vi "enumerateStaticDependencies.vi"(8 "error in (no error)":errorcluster, 11 "SMO.A":refnum<class "SMO.A.lvclass">) -> (0 "error out":errorcluster, 2 "Static Dependencies":refnum<class "SMODependency.lvclass">[](array[class]), 3 "SMO.A out":refnum<class "SMO.A.lvclass">)   [LabVIEW 2013, in "SMO.A.lvclass"]
uses:
  SMO.A.lvclass
  src/Dependency/SMODependency.lvclass
  src/SMO/SMO.lvclass
panel:
  # "For instructions on how to use the JKI State Machine Objects, examples and video tutorials, visit:\nhttp://jki.net/state-machine-objects/\n\nJKI State Machine Objects™\nhttp://jki.net/state-machine-objects/\nCopyright (C) 2005-2015, JKI <info@jki.net>\nALL RIGHTS RESERVED"
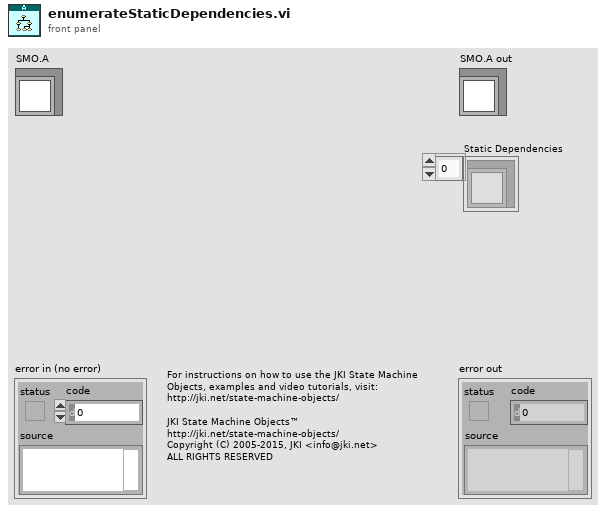
[diagram p1: front panel]
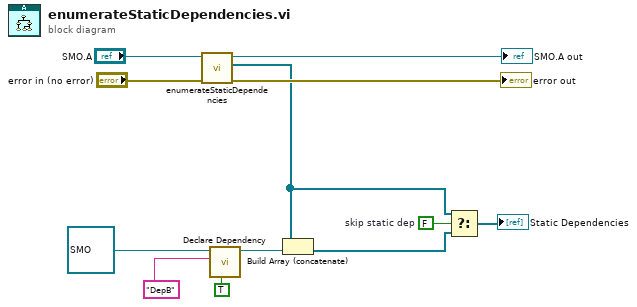
[diagram p0: block diagram]
diagram:
  w5 = FALSE  # skip static dep
  n1 = call-parent "enumerateStaticDependencies.vi"("error in (no error)"="error in (no error)", "SMO"="SMO.A") -> ("error out"=→"error out":errorcluster, "Static Dependencies"=w4:refnum<class "SMODependency.lvclass">[], "SMO out"=→"SMO.A out":refnum<class "SMO.A.lvclass">)  [unwired: 7 in]
  n2 = call "Declare Dependency.vi"("Shared Resource (F)"=TRUE, "Name"="DepB", "Type"=refnum<class "SMO.lvclass"> refnum ("SMO.lvclass")) -> ("Dependency out"=w6:refnum<class "SMODependency.lvclass">)  [unwired: 7 in, 1 out]
  n3 = Build Array (concatenate)(w4, w6) -> (w2:refnum<class "SMODependency.lvclass">[])
  n4 = Select(t=w4, s=w5, f=w2) -> (s? t:f=→"Static Dependencies":refnum<class "SMODependency.lvclass">[])
